vi "Read Geometry Definition.vi"(8 "error in":errorcluster, 9 "Feature":string, 10 "Part":string, 11 "Config Location":path) -> (0 "error out":errorcluster, 2 "Feature Coordinates":refnum<class "Vec3d Class.lvclass">)   [LabVIEW 2011]
uses:
  Vec3d Class/Vec3d Class.lvclass
  <vilib>/Utility/config.llb/Read Key (String).vi
  <vilib>/Utility/config.llb/NI_LVConfig.lvlib
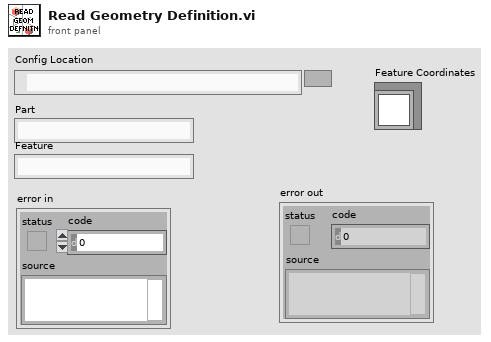
[diagram p1: front panel]
types:
  T1 = typedef "NI_LVConfig.lvlib/Config Data RefNum.ctl" = refnum<k1>
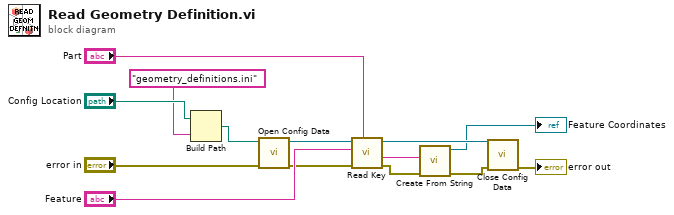
[diagram p0: block diagram]
diagram:
  n1 = Build Path(base path="Config Location", name or relative path="geometry_definitions.ini") -> (appended path=w12:path)
  n2 = call <vilib>:"Open Config Data.vi"("error in (no error)"="error in", "configuration file path"=w12) -> ("error out"=w7:errorcluster, "refnum"=w10:T1)  [unwired: 7 in, 1 out]
  n3 = call-poly <vilib>:"Read Key.vi"("section"="Part", "error in (no error)"=w7, "key"="Feature", "refnum"=w10) -> ("error out"=w5:errorcluster, "value"=w6:string, "refnum out"=w4:T1)  [unwired: 4 in, 1 out]
  n4 = call "Create From String.vi"("error in (no error)"=w5, "Input String"=w6) -> ("error out"=w3:errorcluster, "Vec3d Class out"=→"Feature Coordinates":refnum<class "Vec3d Class.lvclass">)  [unwired: 8 in]
  n5 = call <vilib>:"Close Config Data.vi"("error in (no error)"=w3, "refnum"=w4) -> ("error out"=→"error out":errorcluster)  [unwired: 8 in, 1 out]
